vi "Zarlink Telemetry.vi"(6 "Transceive Delay mS":dbl min=0.0 max=10000.0 step=1.0, 7 "EXID":u32 step=1 format="%.0x", 8 "Parameters":string, 9 "CP_DATA IN":u8[](array[numeric]), 10 "Function":T2(ring), 11 "Command":T1) -> (0 "Data":string, 1 "CP_DATA OUT":u8[](array[numeric]), 2 "Response Code":string, 3 "Response Token":string, 4 "tChecksum Valid":bool, 5 "bChecksum Valid":bool)   [LabVIEW 2009]
uses:
  MICS Config.ctl
  Typedef Command List.ctl
panel:
  out "error out":errorcluster
  in  "error in (no error)":errorcluster
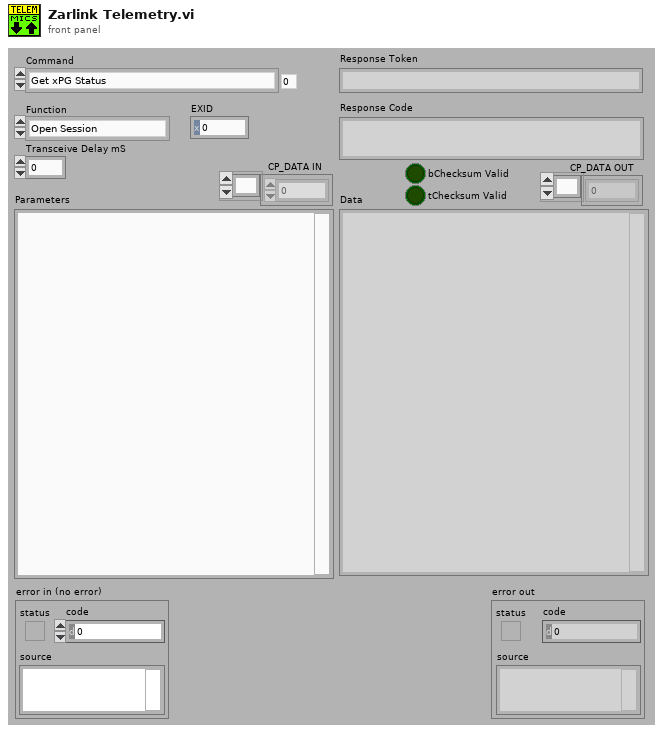
[diagram p1: front panel]
types:
  T1 = typedef "Typedef Command List.ctl" = enum16{"Get xPG Status", "xPG Stimulation", "Select Program", "Increment Program Amplitude", "Decrement Program Amplitude", "Get PoP Constants", "Get PPC Constants", "Get Program Names", "Set Pulse Amplitude", "Increment Pulse Amplitude", "Decrement Pulse Amplitude", "Get Pulse Widths", "Set Pulse Widths", "Increment Pulse Width", "Decrement Pulse Width", "Get Program Frequency", "Set Program Frequency", "Increment Program Frequency", "Decrement Program Frequency", "<reserved 1>", "Charging Control", "Get xPG Identity", "Set xPG Identity", "Restore Program Defaults", "Get Program Definition", "Set Program Definition", "Get Program Constants", "Set Program Constants", "Get Configurable Device Parameters", "Set Configurable Device Parameters", "Get Pulse Constants", "Set Pulse Constants", "Get Lead Limits", "Set Lead Limits", "Get Channel Calibrations", "Set Channel Calibrations", "<reserved 2>", "<reserved 3>", "<reserved 4>", "<reserved 5>", "<reserved 6>", "<reserved 7>", "Get Stim Asic HV Calibrations", "Set Stim Asic HV Calibrations", "<reserved 8>", "<reserved 9>", "Get CP Data", "Set CP Data", "Clear Log", "Read Log", "Append Log", "Get Patient Program Runtime", "Set Patient Program Runtime", "Impedance Measurement", "Enter Storage Mode", "Echo Short", "Echo Long", "Get General Calibration", "Set General Calibration", "Get Trim List", "Set Trim List", "Get Counter", "Set Counter", "Get Test Stimulation", "Set Test Stimulation", "Get Titration Stimulation", "Set Titration Stimulation", "Get Ramp Time", "Set Ramp Time", "Get VBAT", "Set Software Description Block", "Get Software Description Block", "Write Memory", "Read Memory", "Reset xPG", "Erase Flash Block", "Write Vectors", "Read Vectors", "Diagnostic Data", "Set Background Impedance", "Get Background Impedence ", "Undefined"}
  T2 = enum16{"Open Session", "Close Session", "Downlink Only", "Uplink Only", "Transceive (DN -> UP)"}
  T3 = typedef "MICS Config.ctl" = cluster{"flags":cluster{"Auto CCA":u8, "Auto Listen":u8, "Wake-up Mode":u8}, "TransceiverId":cluster{"b3":u8, "b2":u8, "b1":u8}, "CompanyId":u8, "normal":cluster{"chan":u8, "userData":u8, "TxModu":u8, "RxModu":u8, "BlkSize":u8, "maxBlkPerTxPack":u8}, "emergency":cluster{"chan":u8, "userData":u8, "TxModu":u8, "RxModu":u8, "BlkSize":u8, "maxBlkPerTxPack":u8}, "set245GTxdBm":i8, "cal245GTxdBm":i8, "micsRevOnIM":u8, "ccaRssiThreshold":cluster{"ch0":u16, "ch1":u16, "ch2":u16, "ch3":u16, "ch4":u16, "ch5":u16, "ch6":u16, "ch7":u16, "ch8":u16, "ch9":u16}}
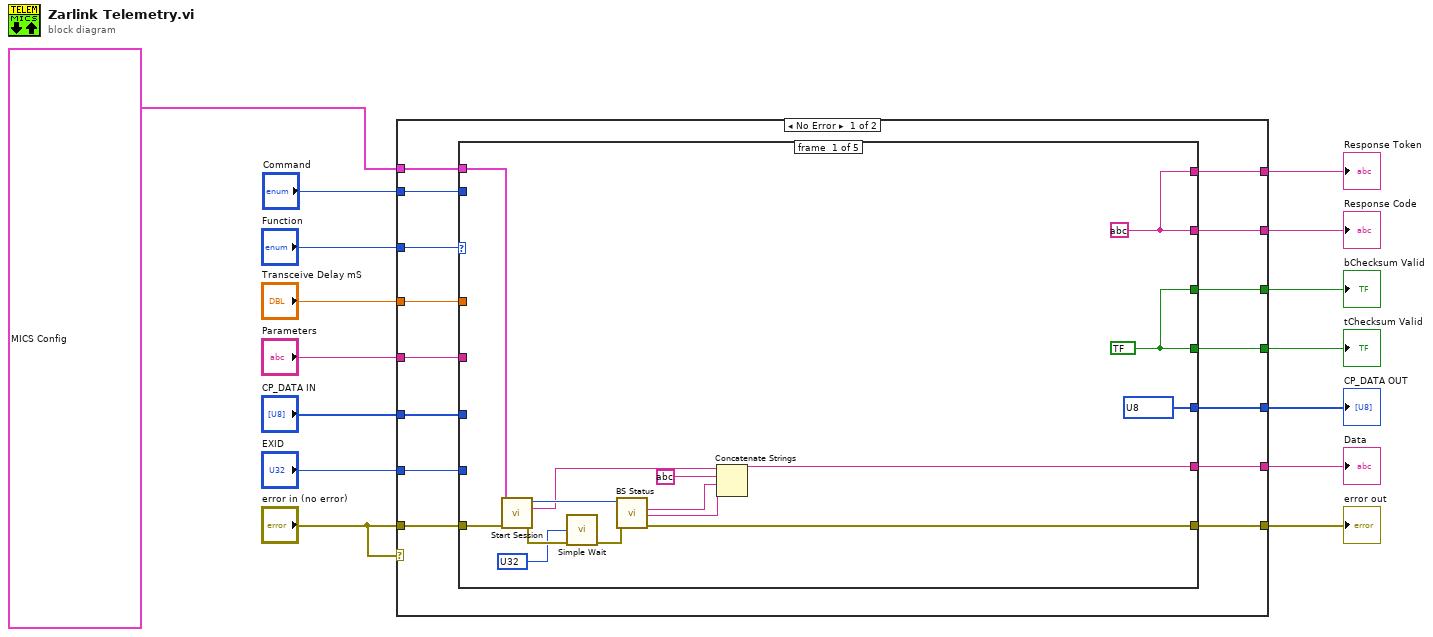
[diagram p0: block diagram]
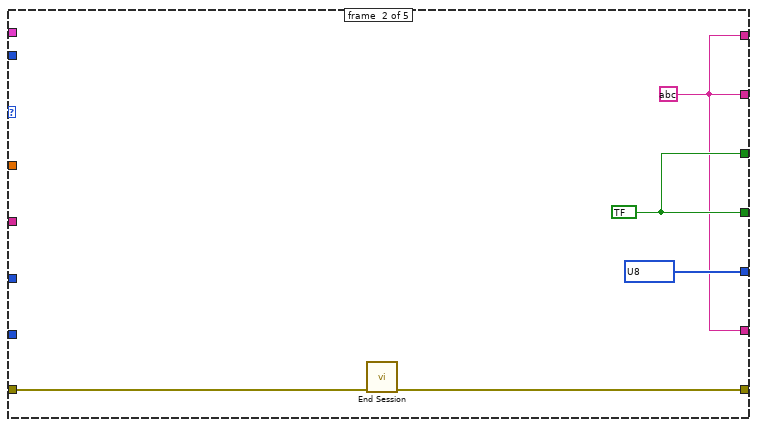
[diagram p2: hidden frame]
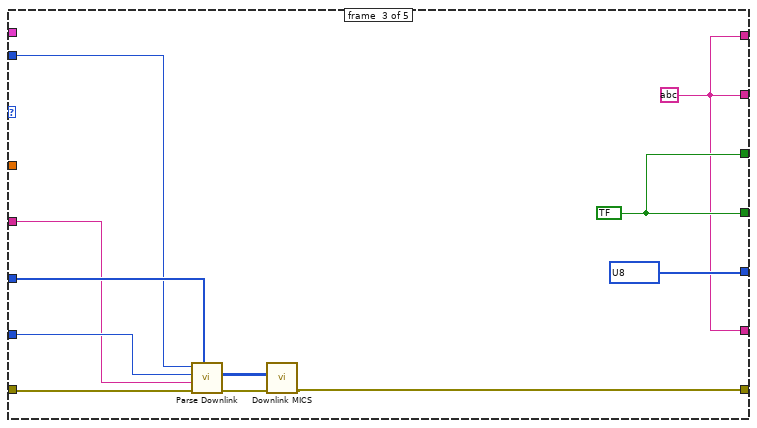
[diagram p3: hidden frame]
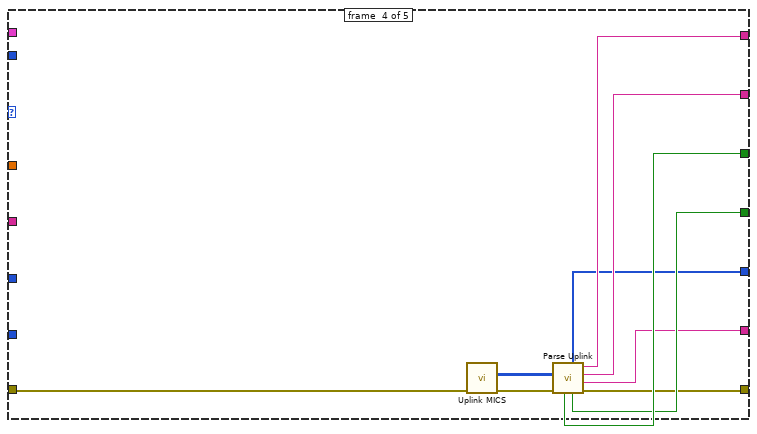
[diagram p4: hidden frame]
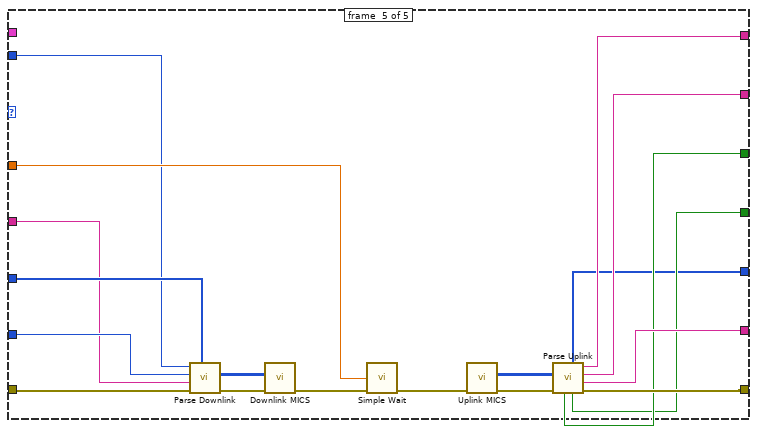
[diagram p5: hidden frame]
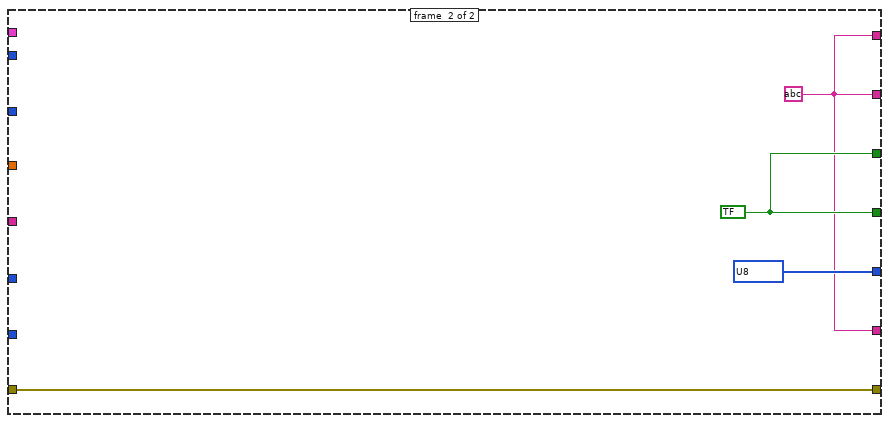
[diagram p6: hidden frame]
diagram:
  n1 = case shown="No Error" "error in (no error)" {
    tunnel: "error in (no error)" -> [w30 w94]
    tunnel: [w29 w94] -> w15
    tunnel: "Function" -> [w28 _]
    tunnel: "Transceive Delay mS" -> [w21 _]
    tunnel: [w22 w91] -> w11
    tunnel: [w23 w91] -> w10
    tunnel: [w24 w93] -> w9
    tunnel: [w25 w93] -> w8
    tunnel: [w26 u8[] ? ("CP_DATA OUT")] -> w7
    tunnel: [w27 w91] -> w6
    tunnel: "CP_DATA IN" -> [w20 _]
    tunnel: "Command" -> [w19 _]
    tunnel: "EXID" -> [w18 _]
    tunnel: "Parameters" -> [w17 _]
    tunnel: T3 ? ("MICS Config Cluster") -> [w16 _]
    frame #0 {
      n2 = case shown="\"Transceive (DN -> UP)\"" w28 {
        tunnel: w30 -> [w45 w48 w59 w62 w88]
        tunnel: [w41 w47 w51 w63 w82] -> w29
        tunnel: [w40 w46 w52 w64 w81] -> w27
        tunnel: [u8[] ? ("CP_DATA OUT") u8[] ? ("CP_DATA OUT") u8[] ? ("CP_DATA OUT") w65 w76] -> w26
        tunnel: [w44 w49 w54 w66 w77] -> w25
        tunnel: [w44 w49 w54 w67 w78] -> w24
        tunnel: [w43 w46 w52 w68 w80] -> w23
        tunnel: [w43 w46 w52 w69 w79] -> w22
        tunnel: w21 -> [_ _ _ _ w90]
        tunnel: w20 -> [_ _ w57 _ w87]
        tunnel: w19 -> [_ _ w55 _ w86]
        tunnel: w18 -> [_ _ w58 _ w85]
        tunnel: w17 -> [_ _ w56 _ w84]
        tunnel: w16 -> [w39 _ _ _ _]
        frame #0 {
          w43 = string ?
          w44 = bool ?
          n3 = call "Start Session.vi"("Error In"=w45, "MICS Config Cluster"=w39) -> ("Error Out"=w33:errorcluster, "Base station info"=w36:string, "Reference Out"=w37:i32)  [unwired: 7 in]
          n4 = call "Simple Wait.vi"("mS"=u32 ?, "error in"=w33) -> ("error out"=w32:errorcluster)  [unwired: 12 in, 1 out]
          n5 = call <vilib>:"BS Status.vi"("Error In"=w32, "Reference In"=w37) -> ("Error Out"=w41:errorcluster, "micsStatus"=w38:string, "flags"=w35:string)  [unwired: 5 in, 1 out]
          n6 = Concatenate Strings(w36, string ?, w35, w38) -> (w40:string)
        }
        frame #1 {
          w46 = string ?
          w49 = bool ?
          n7 = call "End Session.vi"("Error In"=w48) -> ("Error Out"=w47:errorcluster)  [unwired: 10 in]
        }
        frame #2 {
          w52 = string ?
          w54 = bool ?
          n8 = call "Parse Downlink.vi"("CP_DATA IN"=w57, "error in (no error)"=w59, "Parameters"=w56, "EXID"=w58, "Command"=w55) -> ("error out"=w61:errorcluster, "Downlink"=w60:u8[][])  [unwired: 5 in]
          n9 = call "Downlink MICS.vi"("Error In"=w61, "Downlink"=w60) -> ("Error Out"=w51:errorcluster)  [unwired: 8 in, 1 out]
        }
        frame #3 {
          n10 = call "Uplink MICS.vi"("Error In"=w62) -> ("Error Out"=w71:errorcluster, "Uplink"=w70:u8[][])  [unwired: 8 in, 1 out]
          n11 = call "Parse Uplink.vi"("error in (no error)"=w71, "Uplink"=w70) -> ("error out"=w63:errorcluster, "Data"=w64:string, "Response Code"=w68:string, "Response Token"=w69:string, "tChecksum Valid"=w66:bool, "CP_DATA"=w65:u8[], "bChecksum Valid"=w67:bool)  [unwired: 3 in]
        }
        frame #4 {
          n12 = call "Parse Downlink.vi"("CP_DATA IN"=w87, "error in (no error)"=w88, "Parameters"=w84, "EXID"=w85, "Command"=w86) -> ("error out"=w89:errorcluster, "Downlink"=w74:u8[][])  [unwired: 5 in]
          n13 = call "Downlink MICS.vi"("Error In"=w89, "Downlink"=w74) -> ("Error Out"=w73:errorcluster)  [unwired: 8 in, 1 out]
          n14 = call "Simple Wait.vi"("mS"=w90, "error in"=w73) -> ("error out"=w72:errorcluster)  [unwired: 12 in, 1 out]
          n15 = call "Uplink MICS.vi"("Error In"=w72) -> ("Error Out"=w83:errorcluster, "Uplink"=w75:u8[][])  [unwired: 8 in, 1 out]
          n16 = call "Parse Uplink.vi"("error in (no error)"=w83, "Uplink"=w75) -> ("error out"=w82:errorcluster, "Data"=w81:string, "Response Code"=w80:string, "Response Token"=w79:string, "tChecksum Valid"=w77:bool, "CP_DATA"=w76:u8[], "bChecksum Valid"=w78:bool)  [unwired: 3 in]
        }
      }
    }
    frame #1 {
      w91 = string ?
      w93 = bool ?
    }
  }
  "error out" <- w15
  "Response Token" <- w11
  "Response Code" <- w10
  "Data" <- w6
  "CP_DATA OUT" <- w7
  "tChecksum Valid" <- w8
  "bChecksum Valid" <- w9
